vi "LM function and gradient.vi"(6 "output control":T1, 7 "model function":T2, 8 "error in (no error)":errorcluster, 10 "X":dbl[](array[numeric]), 11 "a":dbl[](array[numeric])) -> (0 "error out":errorcluster, 1 "number of function calls":i32, 2 "gradient":dbl[][](array[numeric]), 3 "f(X)":dbl[](array[numeric]))   [LabVIEW 2017, in "NI_Gmath.lvlib"]
uses:
  NI_Gmath.lvlib
  LM model function.ctl
  LM model function reference.ctl
  LM_output select.ctl
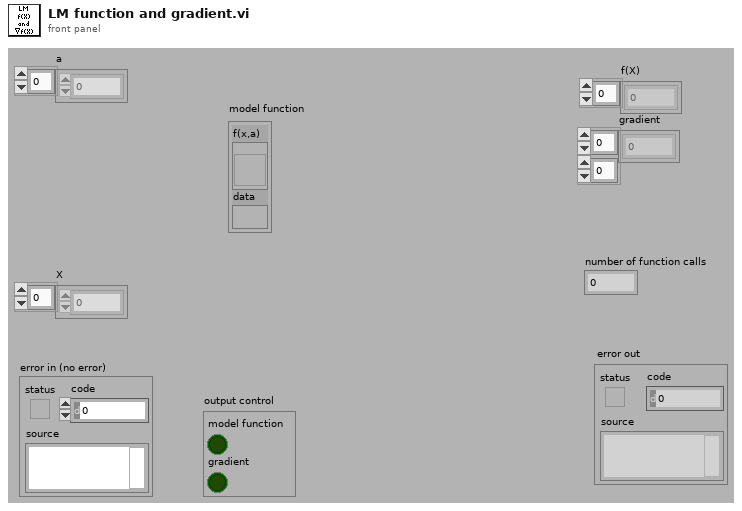
[diagram p1: front panel]
types:
  T1 = typedef "NI_Gmath.lvlib/LM_output select.ctl" = cluster{"model function":bool, "gradient":bool}
  T2 = typedef "NI_Gmath.lvlib/LM model function.ctl" = cluster{"f(x,a)":T3, "data":variant}
  T3 = typedef "NI_Gmath.lvlib/LM model function reference.ctl" = refnum<vi>
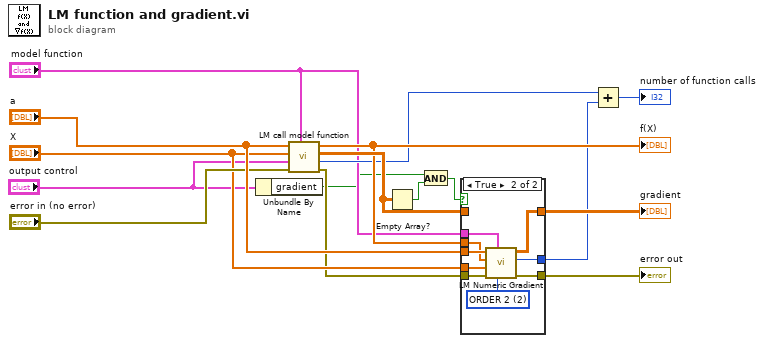
[diagram p0: block diagram]
diagram:
  n1 = Unbundle By Name("output control") -> ("gradient"=w3:bool)
  n2 = call "LM call model function.vi"("model function"="model function", "error in (no error)"="error in (no error)", "output control"="output control", "X"="X", "a"="a") -> ("error out"=w7:errorcluster, "number of function evaluations"=w6:i32, "f'(X,a)"=w16:dbl[][], "f(X)"=w12:dbl[])  [unwired: 3 in]
  "f(X)" <- w12
  n3 = Empty Array?(array=w16) -> (empty?=w2:bool)
  n4 = And(x=w3, y=w2) -> (x .and. y?=w1:bool)
  n5 = case shown="True" w1 {
    tunnel: "a" -> [_ w27]
    tunnel: w12 -> [_ w20]
    tunnel: "model function" -> [_ w26]
    tunnel: w7 -> [w17 w25]
    tunnel: [w18 w21] -> w11
    tunnel: [w17 w24] -> w10
    tunnel: [_ w23] -> w8
    tunnel: "X" -> [_ w22]
    tunnel: w16 -> [w18 _]
    frame False {
    }
    frame True {
      w19 = 2 items=["ORDER 1"=1, "ORDER 2"=2, "ORDER 4"=4] ("order")
      n6 = call "LM Numeric Gradient.vi"("order"=w19, "model function"=w26, "error in (no error)"=w25, "X"=w22, "f(X)"=w20, "a"=w27) -> ("error out"=w24:errorcluster, "number of function evaluations"=w23:i32, "gradient"=w21:dbl[][])  [unwired: 3 in]
    }
  }
  "gradient" <- w11
  "error out" <- w10
  n7 = Add(x=w6, y=w8) -> (x+y=→"number of function calls":i32)
